vi "ex_TCP Query.vi"(0 "TCP Network Connection in":refnum<k5>, 2 "Termination character":string="\n", 7 "Query string":string, 11 "error in (no error)":errorcluster, 12 "Initial byte timeout ms (1000)":i32=1000) -> (4 "TCP Network Connection out":refnum<k5>, 8 "Message data out":string, 10 "Warning":bool, 15 "error out":errorcluster)   [LabVIEW 2013]
doc: "Query and Read will issue a query string over TCP Write, then attempt to retrieve the responce message with minimal recovery time in case of dropped connections/unexpected message lengths.\n\nShould be tweaked to suit expected communicaton specifics.."
panel:
  out "substring":string
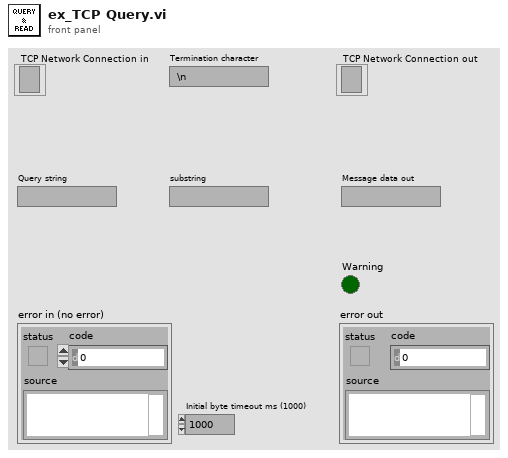
[diagram p1: front panel]
types:
  T1 = enum16{"Standard", "Buffered", "CRLF", "Immediate"}
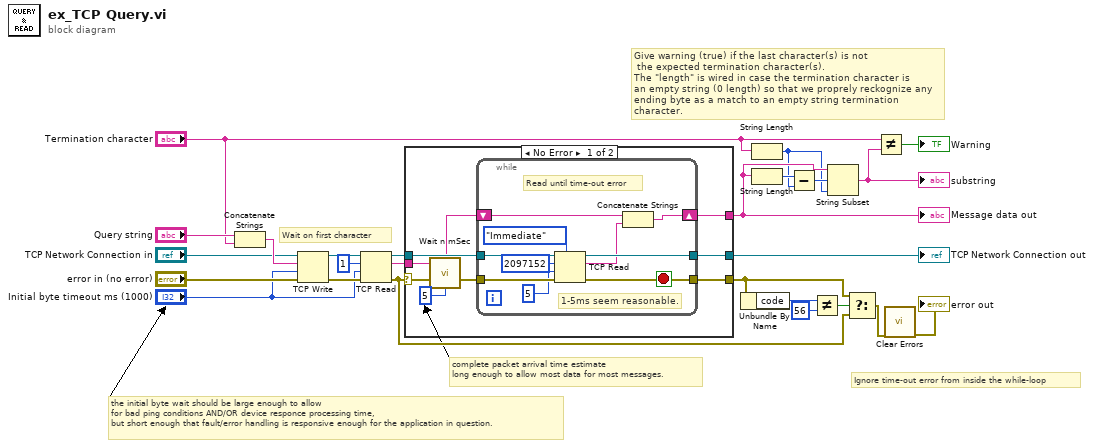
[diagram p0: block diagram]
diagram:
  # "the initial byte wait should be large enough to allow\nfor bad ping conditions AND/OR device responce processing time,\nbut short enough that fault/error handling is responsive enough for the application in question."
  # "complete packet arrival time estimate \nlong enough to allow most data for most messages."
  # "Ignore time-out error from inside the while-loop"
  # "Give warning (true) if the last character(s) is not\n the expected termination character(s).\nThe \"length\" is wired in case the termination character is\nan empty string (0 length) so that we proprely reckognize any\nending byte as a match to an empty string termination character."
  # "Wait on first character"
  n1 = Concatenate Strings("Query string", "Termination character") -> (w25:string)
  n2 = TCP Write(connection ID="TCP Network Connection in", data in=w25, error in (no error)="error in (no error)", 9:"Initial byte timeout ms (1000)") -> (connection ID out=w18:refnum<k5>, error out=w19:errorcluster)  [unwired: 1 out]
  n3 = TCP Read(connection ID=w18, bytes to read=1, error in (no error)=w19, 9:"Initial byte timeout ms (1000)") -> (connection ID out=w17:refnum<k5>, data out=w16:string, error out=w7:errorcluster)  [unwired: 1 in]
  n4 = case shown="No Error" w7 {
    selector: w7 -> [w26 w44]
    tunnel: [w33 w46] -> w23
    tunnel: [w32 w44] -> w8
    tunnel: w17 -> [w31 w46]
    tunnel: w16 -> [w28 w45]
    tunnel: [w27 w45] -> w15
    frame No Error {
      n5 = call "Wait n mSec.vi"("Error in (no error)"=w26, "Milliseconds to Wait (1)"=u32 5) -> ("Error Out"=w30:errorcluster)  [unwired: 13 in]
      n6 = while {
        tunnel: [w43] -> w33
        tunnel: [w35] -> w32
        tunnel: w31 -> [w41]
        tunnel: w30 -> [w40]
        shift-right: [w36] -> w27
        shift-left: w28 -> [w38]
        stop <- w35 stop-if-true
        # "1-5ms seem reasonable."
        # "Read until time-out error"
        n7 = TCP Read(connection ID=w41, bytes to read=2097152, error in (no error)=w40, 7:T1."Immediate" ("mode (standard)"), 9:5 ("timeout ms (25000)")) -> (connection ID out=w43:refnum<k5>, data out=w37:string, error out=w35:errorcluster)
        n8 = Concatenate Strings(w38, w37) -> (w36:string)
      }
    }
    frame Error {
    }
  }
  "Message data out" <- w15
  "TCP Network Connection out" <- w23
  n9 = Unbundle By Name(w8) -> ("code"=w11:i32)
  n10 = String Length(string="Termination character") -> (length=w3:i32)
  n11 = String Length(string=w15) -> (length=w6:i32)
  n12 = Subtract(x=w6, y=w3) -> (x-y=w4:i32)
  n13 = Not Equal?(x=w11, y=56) -> (x != y?=w9:bool)
  n14 = String Subset(string=w15, offset (0)=w4, length (rest)=w3) -> (substring=w13:string)
  "substring" <- w13
  n15 = Select(t=w8, s=w9, f=w7) -> (s? t:f=w2:errorcluster)
  n16 = Not Equal?(x="Termination character", y=w13) -> (x != y?=→"Warning":bool)
  n17 = call <vilib>:"Clear Errors.vi"("error in (no error)"=w2) -> ("error out"=→"error out":errorcluster)  [unwired: 6 in]
